vi "Routine.vi"(8 "error in (no error)":errorcluster, 11 "Node Ptr":T1 format="%.0x") -> (0 "error out":errorcluster)   [LabVIEW 2015, in "Diagnostics Addon System Explorer.lvlib"]
uses:
  Diagnostics Addon System Explorer.lvlib
  <vilib>/NI Veristand/Custom Device API/Custom Device Item Ref.ctl
  Shared/FG Action.ctl
  Shared/GUID Lookup.vi
  <vilib>/NI Veristand/Custom Device API/NI VeriStand - Set Item Property.vi
  <vilib>/NI Veristand/Custom Device API/Set Item Property (U32).vi
  <vilib>/NI Veristand/Custom Device API/NI VeriStand - Get Item Property.vi
  <vilib>/NI Veristand/Custom Device API/Get Item Property (U32).vi
  <vilib>/NI Veristand/Custom Device API/Custom Device API.lvlib
panel:
  in  "ID":u16 format="%.0x"
  in  "Description":string
  in  "Name":string
  in  "SHDocVw.IWebBrowser":refnum<k7>(container)
  in  "Header":cluster{"Section Name":string}={"Section Name"="Custom Device Item Settings"}
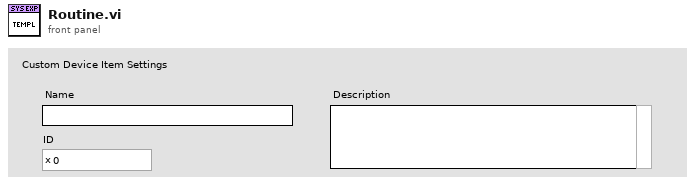
[diagram p1: front panel]
types:
  T1 = typedef "Custom Device API.lvlib/Custom Device Item Ref.ctl" = u64
  T2 = typedef "Diagnostics Addon System Explorer.lvlib/FG Action.ctl" = enum16{"Get", "Set"}
  T3 = typedef "Custom Device API.lvlib/Custom Device Item Info.ctl" = cluster{"Name":string, "Is Channel":bool, "GUID":string, "Is Waveform":bool}
  T4 = typedef "Custom Device API.lvlib/Custom Device Commands.ctl" = enum16{"Default", "Item renamed", "Shutdown", "Dynamic button pressed"}
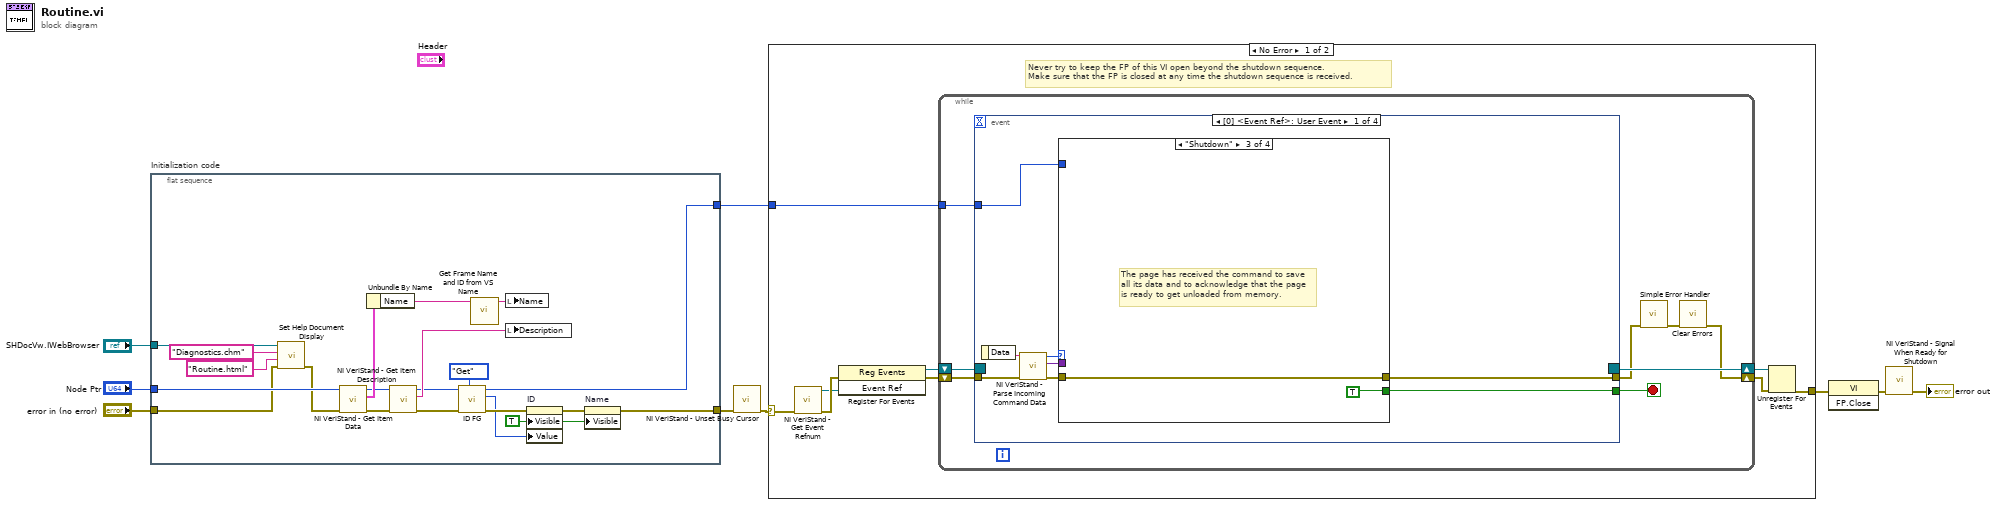
[diagram p0: block diagram]
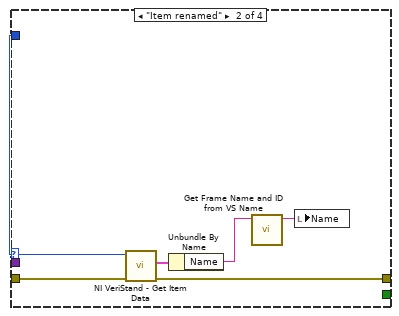
[diagram p3: hidden frame]
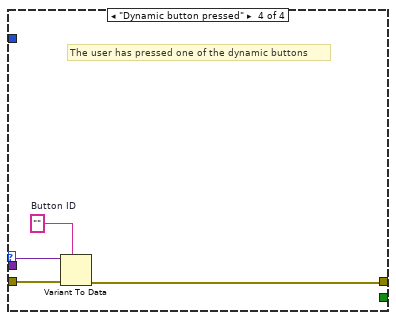
[diagram p4: hidden frame]
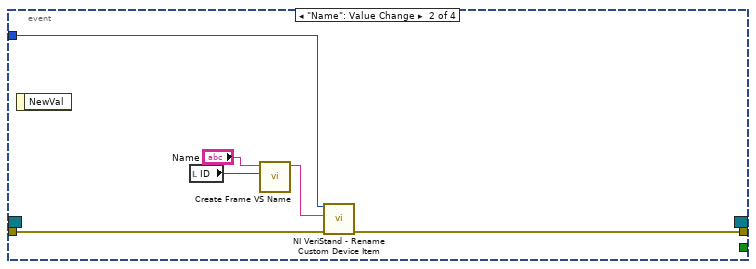
[diagram p5: hidden frame]
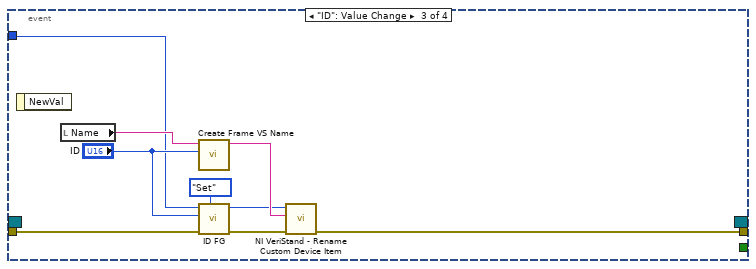
[diagram p6: hidden frame]
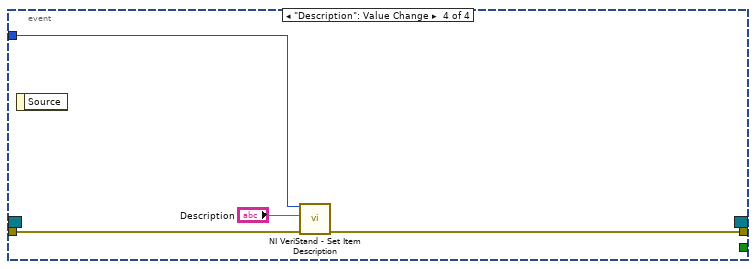
[diagram p7: hidden frame]
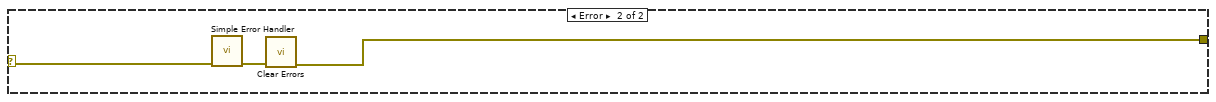
[diagram p8: hidden frame]
diagram:
  n1 = flat-sequence "Initialization code" {
    tunnel: "error in (no error)" -> [w11]
    tunnel: "Node Ptr" -> [w21]
    tunnel: [w12] -> w5
    tunnel: [w19] -> w2
    tunnel: "SHDocVw.IWebBrowser" -> [w20]
    frame #0 {
      w14 = TRUE ("Visible")
      n2 = call "Set Help Document Display.vi"("error in (no error)"=w11, "HTML File"="Routine.html", "Main CHM File"="Diagnostics.chm", "SHDocVw.IWebBrowser2"=w20) -> ("error out"=w10:errorcluster)  [unwired: 7 in]
      n3 = call <vilib>:"NI VeriStand - Get Item Data.vi"("error in (no error)"=w10, "Item Ref in"=w21) -> ("error out"=w22:errorcluster, "Item Info"=w29:T3, "Item Ref out"=w23:T1)  [unwired: 7 out]
      n4 = Unbundle By Name(w29) -> ("Name"=w27:string)
      n5 = call <vilib>:"NI VeriStand - Get Item Description.vi"("error in (no error)"=w22, "Item Ref in"=w23) -> ("error out"=w25:errorcluster, "Description"=w30:string, "Item Ref out"=w24:T1)  [unwired: 7 out]
      n6 = call "ID FG.vi"("Action"=FG_Action."Get", "error in (no error)"=w25, "Device Item Ref in"=w24) -> ("error out"=w17:errorcluster, "ID"=w16:u32, "Device Item Ref out"=w19:T1)  [unwired: 6 in]
      n7 = call "Get Frame Name and ID from VS Name.vi"("VS PID Name"=w27) -> ("PID Name"=w26:string)  [unwired: 9 in, 1 out]
      n8 = local write "Name"(w26) -> ()
      n9 = local write "Description"(w30) -> ()
      n10 = property on="ID" class="DigNum (strict)"(error in=w17, "Visible"=w14, "Value"=w16) -> (error out=w15:errorcluster)  [unwired: 1 in, 1 out]
      n11 = property on="Name" class="Str"(error in=w15, "Visible"=w14) -> (error out=w12:errorcluster)  [unwired: 1 in, 1 out]
    }
  }
  n12 = call <vilib>:"NI VeriStand - Unset Busy Cursor.vi"("error in (no error)"=w5) -> ("error out"=w4:errorcluster)  [unwired: 10 out]
  n13 = case shown="No Error" w4 {
    selector: w4 -> [w31 w90]
    tunnel: [w36 w88] -> w9
    tunnel: w2 -> [w32 _]
    frame No Error {
      # "Never try to keep the FP of this VI open beyond the shutdown sequence.\nMake sure that the FP is closed at any time the shutdown sequence is received."
      n14 = call <vilib>:"NI VeriStand - Get Event Refnum.vi"("error in (no error)"=w31) -> ("error out"=w39:errorcluster, "Event Ref"=w35:refnum<user-event>)  [unwired: 9 out]
      n15 = register-events(error in=w39, w35) -> (reference out=w33:refnum<event-registration>, error out=w34:errorcluster)  [unwired: 1 in]
      n16 = while {
        tunnel: w32 -> [w43]
        shift-right: [w40] -> w37
        shift-left: w34 -> [w46]
        shift-right: [w47] -> w38
        shift-left: w33 -> [w45]
        stop <- w44 stop-if-true
        n17 = event shown="[0] <Event Ref>: User Event" {
          selector: w45 -> [_ _ _ _]
          dyn-events: [_ _ _ _] -> w47
          timeout: _ -> [_ _ _ _]
          tunnel: w46 -> [w55 w74 w80 w86]
          tunnel: [w51 _ _ _] -> w44
          tunnel: [w50 w73 w82 w85] -> w42
          tunnel: w43 -> [w49 w72 w77 w87]
          event User Event {
            n18 = event-data() -> ("Data"=w54:string)  [unwired: 1 out]
            n19 = call <vilib>:"NI VeriStand - Parse Incoming Command Data.vi"("error in (no error)"=w55, "Incoming data"=w54) -> ("error out"=w53:errorcluster, "Outgoing data"=w48:variant, "Action"=w52:T4)  [unwired: 7 out]
            n20 = case shown="\"Shutdown\"" w52 {
              tunnel: w53 -> [w56 w62 w63 w68]
              tunnel: [_ _ TRUE _] -> w51
              tunnel: [w56 w59 w63 w65] -> w50
              tunnel: w49 -> [_ w61 _ _]
              tunnel: w48 -> [_ _ _ w67]
              frame "Default", Default {
              }
              frame "Item renamed" {
                n21 = call <vilib>:"NI VeriStand - Get Item Data.vi"("error in (no error)"=w62, "Item Ref in"=w61) -> ("error out"=w59:errorcluster, "Item Info"=w60:T3)  [unwired: 8 out]
                n22 = Unbundle By Name(w60) -> ("Name"=w58:string)
                n23 = call "Get Frame Name and ID from VS Name.vi"("VS PID Name"=w58) -> ("PID Name"=w57:string)  [unwired: 9 in, 1 out]
                n24 = local write "Name"(w57) -> ()
              }
              frame "Shutdown" {
                # "The page has received the command to save all its data and to acknowledge that the page is ready to get unloaded from memory."
              }
              frame "Dynamic button pressed" {
                w66 = ""  # Button ID
                # "The user has pressed one of the dynamic buttons"
                n25 = Variant To Data(error in=w68, type=w66, Variant=w67) -> (error out=w65:errorcluster)  [unwired: 1 out]
              }
            }
          }
          event "Name": Value Change {
            n26 = event-data() -> ()  [unwired: 2 out]
            n27 = local read "ID"() -> (w71:u16)
            n28 = call "Create Frame VS Name.vi"("PID Number"=w71, "PID Name"="Name") -> ("VS Name"=w69:string)  [unwired: 9 in]
            n29 = call <vilib>:"NI VeriStand - Rename Custom Device Item.vi"("error in (no error)"=w74, "New Name"=w69, "Item Ref in"=w72) -> ("error out"=w73:errorcluster)  [unwired: 1 in, 7 out]
          }
          event "ID": Value Change {
            n30 = event-data() -> ()  [unwired: 2 out]
            n31 = local read "Name"() -> (w81:string)
            n32 = call "Create Frame VS Name.vi"("PID Number"="ID", "PID Name"=w81) -> ("VS Name"=w83:string)  [unwired: 9 in]
            n33 = call "ID FG.vi"("Action"=FG_Action."Set", "error in (no error)"=w80, "ID"="ID", "Device Item Ref in"=w77) -> ("error out"=w79:errorcluster, "Device Item Ref out"=w76:T1)  [unwired: 5 in, 1 out]
            n34 = call <vilib>:"NI VeriStand - Rename Custom Device Item.vi"("error in (no error)"=w79, "New Name"=w83, "Item Ref in"=w76) -> ("error out"=w82:errorcluster)  [unwired: 1 in, 7 out]
          }
          event "Description": Value Change {
            n35 = event-data() -> ()  [unwired: 2 out]
            n36 = call <vilib>:"NI VeriStand - Set Item Description.vi"("error in (no error)"=w86, "Description"="Description", "Item Ref in"=w87) -> ("error out"=w85:errorcluster)  [unwired: 8 out]
          }
        }
        n37 = call <vilib>:"Simple Error Handler.vi"("error in (no error)"=w42) -> ("error out"=w41:errorcluster)  [unwired: 1 in, 7 out]
        n38 = call <vilib>:"Clear Errors.vi"("error in (no error)"=w41) -> ("error out"=w40:errorcluster)  [unwired: 1 in, 5 out]
      }
      n39 = Unregister For Events(event registration refnum=w38, error in=w37) -> (error out=w36:errorcluster)
    }
    frame Error {
      n40 = call <vilib>:"Simple Error Handler.vi"("error in (no error)"=w90) -> ("error out"=w89:errorcluster)  [unwired: 1 in, 7 out]
      n41 = call <vilib>:"Clear Errors.vi"("error in (no error)"=w89) -> ("error out"=w88:errorcluster)  [unwired: 1 in, 5 out]
    }
  }
  n42 = invoke class="VI" method="FP.Close"(error in=w9) -> (error out=w8:errorcluster)  [unwired: 2 in, 2 out]
  n43 = call <vilib>:"NI VeriStand - Signal When Ready for Shutdown.vi"("error in (no error)"=w8) -> ("error out"=→"error out":errorcluster)  [unwired: 10 out]
